vi "max (SubVI).vi"(10 "initialized array":dbl[](array[numeric])) -> (2 "y":dbl)   [LabVIEW 2017]
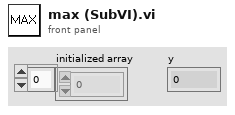
[diagram p1: front panel]
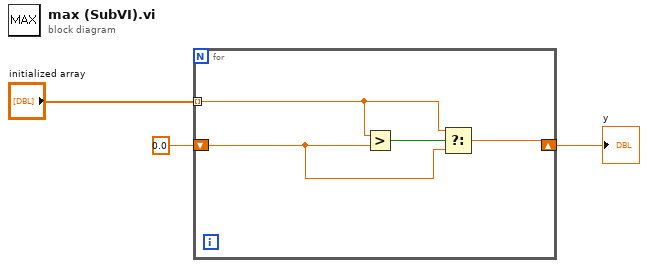
[diagram p0: block diagram]
diagram:
  n1 = for {
    tunnel: "initialized array" -> [w6] mode=indexing
    shift-right: [w4] -> w1
    shift-left: 0.0 ("y") -> [w5]
    n2 = Greater?(x=w6, y=w5) -> (0:w7:bool)
    n3 = Select(t=w6, s=w7, f=w5) -> (s? t:f=w4:dbl)
  }
  "y" <- w1
